vi "Format Item Property Name.vi"(10 "index":i32, 11 "Base Property Name":string) -> (3 "Item Property Name":string)   [LabVIEW 2016]
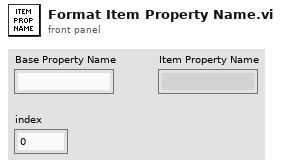
[diagram p1: front panel]
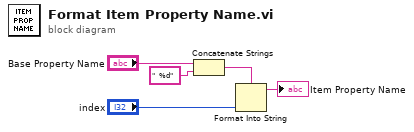
[diagram p0: block diagram]
diagram:
  n1 = Concatenate Strings("Base Property Name", "  %d" ("string")) -> (w4:string)
  n2 = Format Into String(format string=w4, "index") -> (resulting string=→"Item Property Name":string)  [unwired: 2 in, 1 out]
